vi "FPGA Top Level.vi"   [LabVIEW 2017]
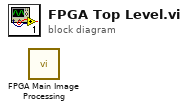
[diagram p0: block diagram]
diagram:
  n1 = call "FPGA Main Image Processing.vi"() -> ()  [unwired: 12 in]
